vi "Dialog_Start (SubVI).vi"() -> ()   [LabVIEW 2017]
uses:
  Global_SNK3_HF.vi
panel:
  out "StringVer":string
  out "String":string
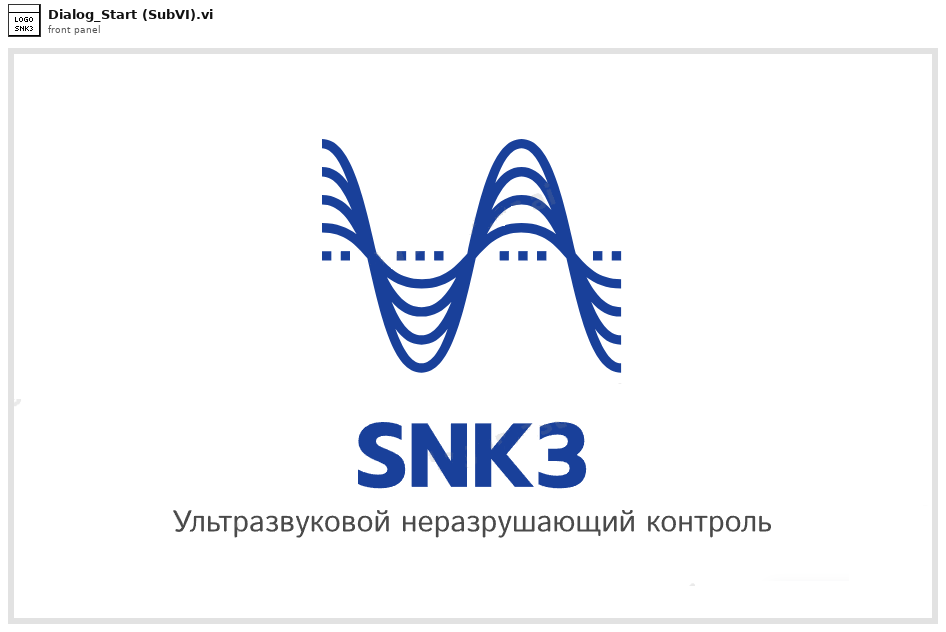
[diagram p1: front panel]
types:
  T1 = cluster{"Версия:":string, "Наименование ПО:":string, "Год выпуска:":string, "Производитель:":string, "MD5":string, "Наименование ПО полное:":string, "Build":string}
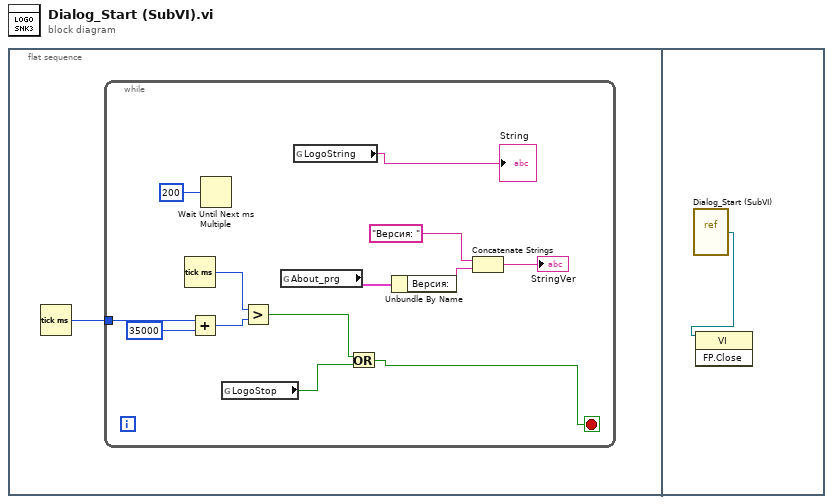
[diagram p0: block diagram]
diagram:
  n1 = flat-sequence {
    frame #0 {
      n2 = Tick Count (ms)() -> (millisecond timer value=w1:u32)
      n3 = while {
        tunnel: w1 -> [w13]
        stop <- w7 stop-if-true
        n4 = Tick Count (ms)() -> (millisecond timer value=w10:u32)
        n5 = Add(x=w13, y=u32 35000) -> (x+y=w11:u32)
        n6 = Wait Until Next ms Multiple(millisecond multiple=u32 200 ("milliseconds to wait")) -> ()  [unwired: 1 out]
        n7 = global read "Global_SNK3_HF.vi" "LogoStop"() -> (w8:bool)
        n8 = Greater?(x=w10, y=w11) -> (0:w9:bool)
        n9 = global read "Global_SNK3_HF.vi" "About_prg"() -> (w6:T1)
        n10 = global read "Global_SNK3_HF.vi" "LogoString"() -> (→"String":string)
        n11 = Or(x=w9, y=w8) -> (x .or. y?=w7:bool)
        n12 = Unbundle By Name(w6) -> ("Версия:"=w5:string)
        n13 = Concatenate Strings("Версия: " ("string"), w5) -> (→"StringVer":string)
      }
    }
    frame #1 {
      n14 = vi-ref "Dialog_Start (SubVI).vi"() -> (w15:refnum<vi>)
      n15 = invoke class="VI" method="FP.Close"(reference=w15) -> ()  [unwired: 2 in, 3 out]
    }
  }
